vi "Mass Compile a Folder.vi"(6 "Append Log?":bool, 8 "error in (no error)":errorcluster, 9 "Log Path":path, 10 "Number of VIs to Cache (100)":u32=100, 11 "Directory Path":path) -> (0 "error out":errorcluster, 3 "User Stopped?":bool)   [LabVIEW 2014, in "SLL Utilities.lvlib"]
doc: "Loads and compiles VIs in a directory, including VIs in subdirectories. \n\nThis method is similar to the Mass Compile option in the Mass Compile dialog box."
uses:
  SLL Utilities.lvlib
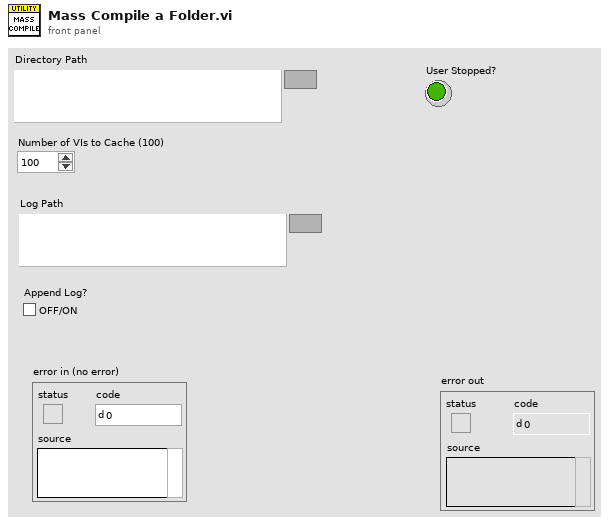
[diagram p1: front panel]
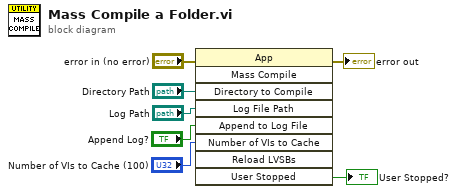
[diagram p0: block diagram]
diagram:
  n1 = invoke class="App" method="Mass Compile"(error in="error in (no error)", "Directory to Compile"="Directory Path", "Log File Path"="Log Path", "Append to Log File"="Append Log?", "Number of VIs to Cache"="Number of VIs to Cache (100)") -> (error out=→"error out":errorcluster, "User Stopped"=→"User Stopped?":bool)  [unwired: 4 in, 7 out]
